vi "Store Plugin Data.vi"(8 "error in (no error)":errorcluster, 11 "Generic Plugin out":refnum<class "Generic Plugin.lvclass">) -> (0 "error out":errorcluster, 3 "output cluster":T1)   [LabVIEW 2011, in "Generic Plugin.lvclass"]
uses:
  Generic Plugin.lvclass
panel:
  in  "pCOMM Ref 2":T1
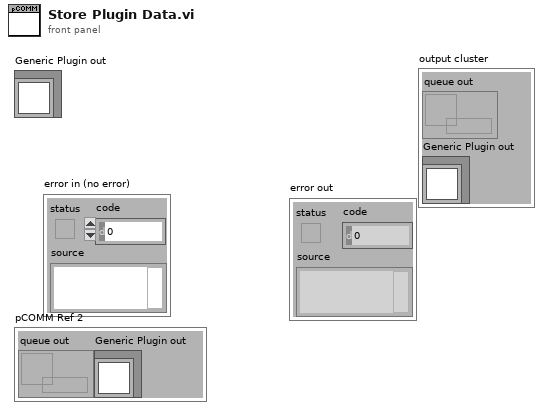
[diagram p1: front panel]
types:
  T1 = cluster{"queue out":refnum<queue>, "Generic Plugin out":refnum<class "Generic Plugin.lvclass">}
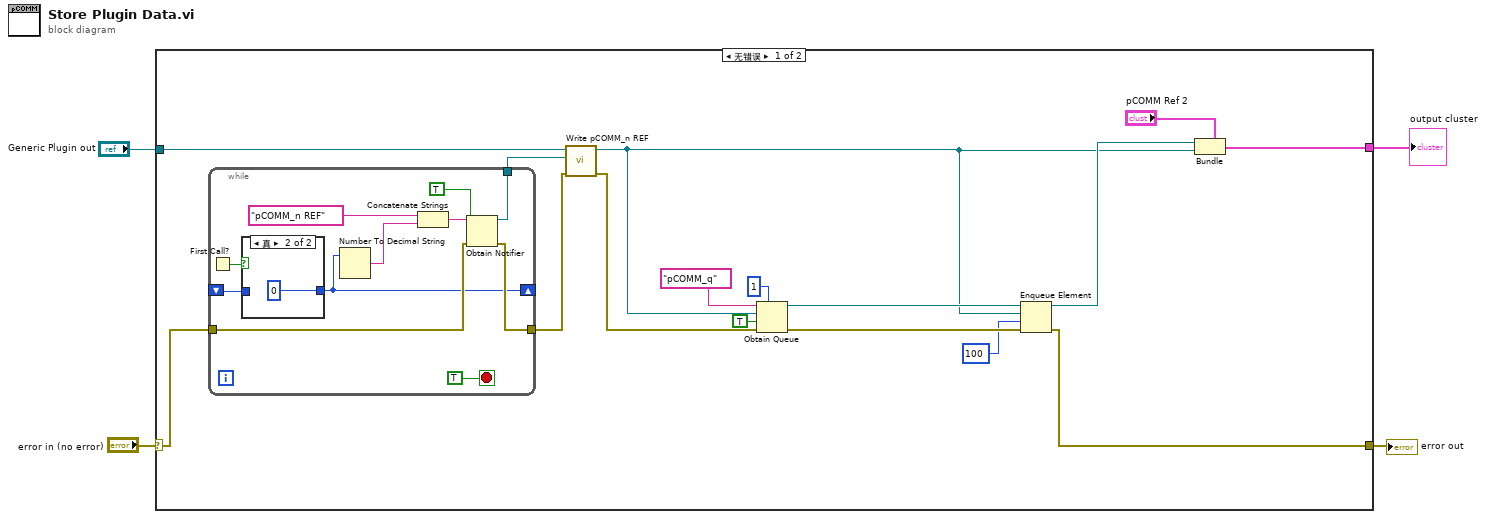
[diagram p0: block diagram]
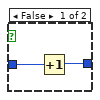
[diagram p2: hidden frame]
diagram:
  n1 = case shown="无错误" "error in (no error)" {
    selector: "error in (no error)" -> [w6 w35]
    tunnel: [w12 w35] -> w4
    tunnel: "Generic Plugin out" -> [w10 _]
    tunnel: [w11 _] -> w1
    frame No Error {
      n2 = while {
        tunnel: [w30] -> w7
        tunnel: w6 -> [w29]
        tunnel: [w28] -> w5
        shift-right: [w24] -> _
        shift-left: _ -> [w26]
        stop <- TRUE stop-if-true
        n3 = First Call?() -> (First Call?: T/F=w25:bool)
        n4 = case shown="真" w25 {
          tunnel: w26 -> [w33 _]
          tunnel: [w32 0] -> w24
          frame False {
            n5 = Increment(x=w33) -> (x+1=w32:i32)
          }
          frame True {
          }
        }
        n6 = Number To Decimal String(number=w24) -> (decimal integer string=w23:string)  [unwired: 1 in]
        n7 = Concatenate Strings("pCOMM_n REF" ("name (unnamed)"), w23) -> (w21:string)
        n8 = Obtain Notifier(name (unnamed)=w21, notification data type=TRUE, error in (no error)=w29) -> (notifier out=w30:refnum<notifier>, error out=w28:errorcluster)  [unwired: 1 in, 1 out]
      }
      n9 = call "Write pCOMM_n REF.vi"("error in (no error)"=w5, "pCOMM_n REF"=w7, "Generic Plugin in"=w10) -> ("error out"=w8:errorcluster, "Generic Plugin out"=w9:refnum<class "Generic Plugin.lvclass">)  [unwired: 7 in]
      n10 = Obtain Queue(max queue size (-1, unlimited)=1, name (unnamed)="pCOMM_q", element data type=w9, create if not found? (T)=TRUE, error in (no error)=w8) -> (queue out=w19:refnum<queue>, error out=w16:errorcluster)  [unwired: 1 out]
      n11 = Enqueue Element(queue=w19, element=w9, timeout in ms (-1)=100, error in (no error)=w16) -> (queue out=w17:refnum<queue>, error out=w12:errorcluster)  [unwired: 1 out]
      n12 = Bundle(cluster="pCOMM Ref 2", "queue out"=w17, "Generic Plugin out"=w9) -> (w11:T1)
    }
    frame Error {
    }
  }
  "error out" <- w4
  "output cluster" <- w1
